vi "Initialise.vi"(8 "error in (no error)":errorcluster, 11 "MsgPackEvents in":refnum<class "MsgPackEvents.lvclass">) -> (0 "error out":errorcluster, 3 "MsgPackEvents out":refnum<class "MsgPackEvents.lvclass">)   [LabVIEW 2020, in "wamplv.lvlib" / "MsgPackEvents.lvclass"]
uses:
  MsgPackEvents.lvclass
  MsgPackEvents.lvclass/MsgPackEvents.ctl
  EventsParent/Events.lvclass
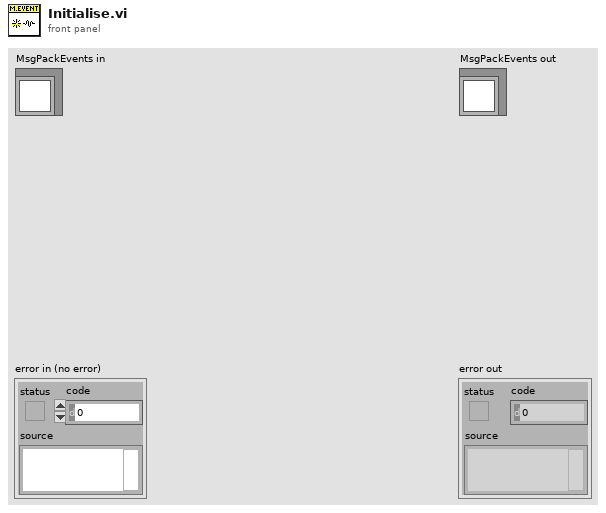
[diagram p1: front panel]
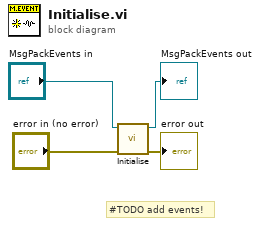
[diagram p0: block diagram]
diagram:
  # "#TODO add events!"
  n1 = call-parent "Initialise.vi"("error in (no error)"="error in (no error)", "EventsParent in"="MsgPackEvents in") -> ("error out"=→"error out":errorcluster, "EventsParent out"=→"MsgPackEvents out":refnum<class "MsgPackEvents.lvclass">)  [unwired: 8 in]
